vi "Periodic Tasks.vi"(8 "error in":errorcluster) -> ()   [LabVIEW 2016]
doc: "This VI runs in parallel to other tasks. It can contain as many user-defined periodic loops as you need. These can carry out PID or other sorts of timed response."
uses:
  <vilib>/Rock Robotics/WPI/DriverStation/WPI_DriverStationRobotMode2.ctl
  <vilib>/Rock Robotics/WPI/Utilities/WPI_GetSetVariantRefNum.vi
  <vilib>/Rock Robotics/Network Tables/NT Write Number.vi
  <vilib>/Instr/_visa.llb/VISA Configure Serial Port (Instr).vi
  Systems/Global 1.vi
  Global 2.vi
panel:
  out "Waveform Chart":dbl(graph)
  out "PSI":dbl=101.0986199
  out "Shoot 0":dbl format="%#_13g"
  out "Shoot 1":dbl format="%#_13g"
  out "read buffer":string="B:2,X:203.00"
  in  "Search_Params":string[](array[string])=["B", "X", "Y", "W1", "H1", "W2", "H2"]
  out "Last Complete Message":string="B:2,X:203.00,Y:125.00,W1:11,H1:27,W2:8,H2:25"
  out "length":i32=44
  in  "off set":dbl format="%#_13g"
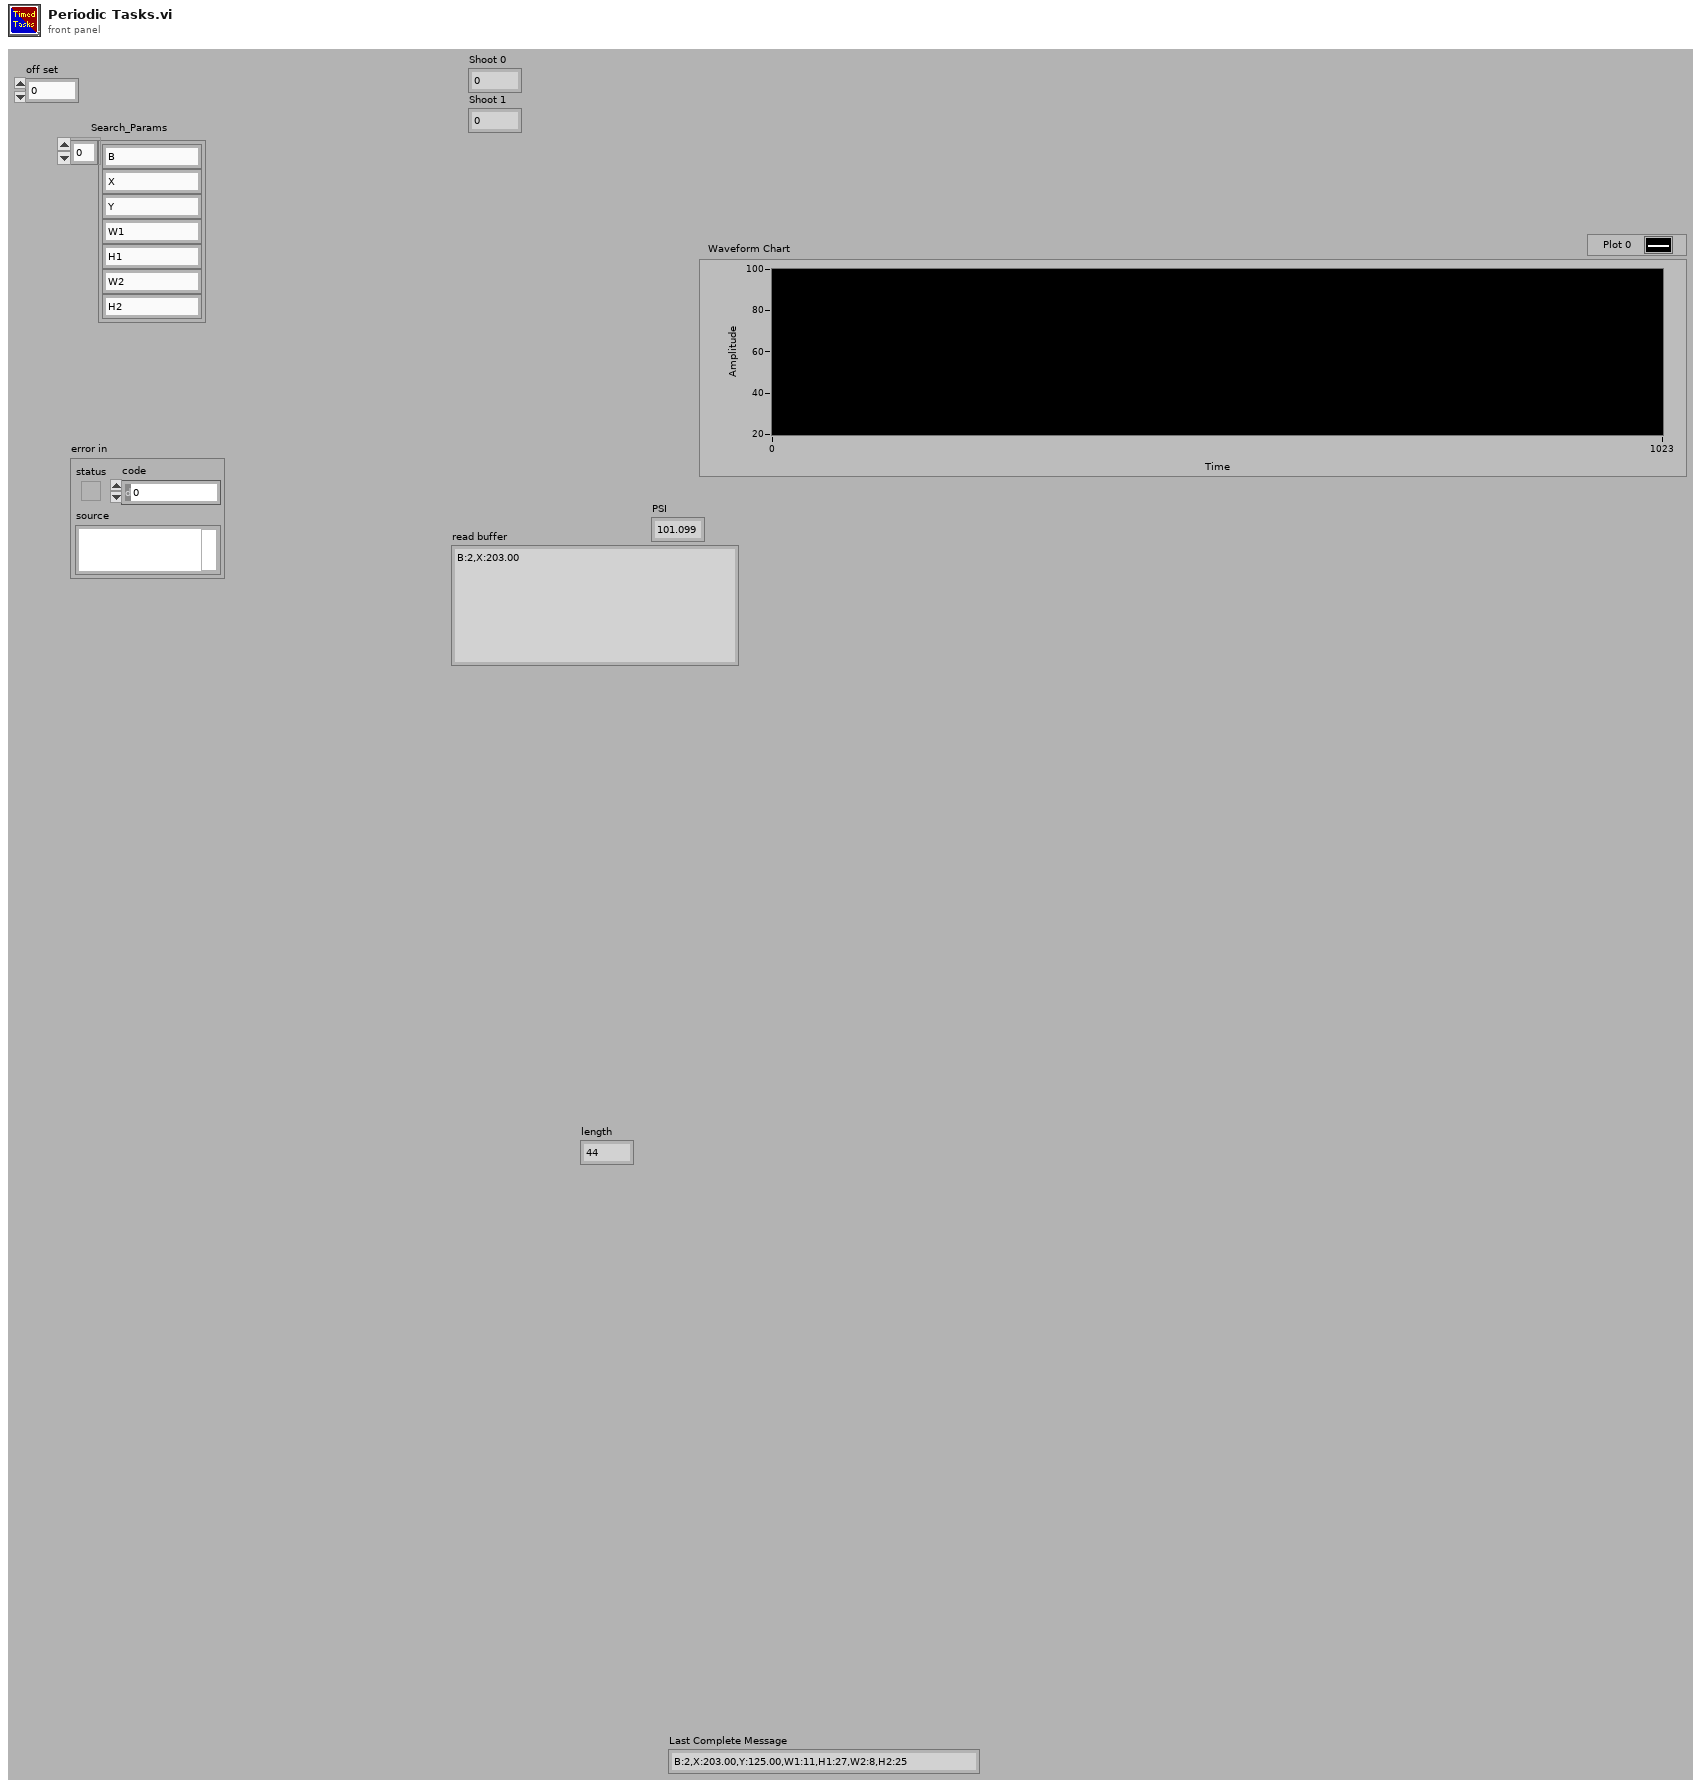
[diagram p1: front panel]
types:
  T1 = typedef "WPI_JoystickDevRef.ctl" = cluster{"Device":T2}
  T2 = typedef "WPI_JoystickDeviceEnum.ctl" = enum16{"USB 0", "USB 1", "USB 2", "USB 3", "USB 4", "USB 5"}
  T3 = typedef "WPI_AnalogChannelDevRef.ctl" = cluster{"DevStatus":errorcluster, "Analog Channel":T4}
  T4 = typedef "FPGA_AIChannel.ctl" = enum8{"AI 0", "AI 1", "AI 2", "AI 3", "AI MXP 0", "AI MXP 1", "AI MXP 2", "AI MXP 3", "Invalid"}
  T5 = typedef "WPI_MotorControlDeviceRef.ctl" = cluster{"DeviceStatus":errorcluster, "Type":T6, "PWM":cluster{"PWM Channel":T7, "DeadBand":T8}, "CAN":cluster{"Device Number":u8, "SetOutput VI Ref":variant, "GetOutput VI Ref":variant, "Enable VI Ref":variant, "Disable VI Ref":variant, "Data":variant}, "Invert":bool}
  T6 = typedef "WPI_MotorControlType.ctl" = enum16{"PWM", "CAN"}
  T7 = typedef "FPGA_DIOPWMChannel.ctl" = enum8{"PWM 0", "PWM 1", "PWM 2", "PWM 3", "PWM 4", "PWM 5", "PWM 6", "PWM 7", "PWM 8", "PWM 9", "PWM MXP 0", "PWM MXP 1", "PWM MXP 2", "PWM MXP 3", "PWM MXP 4", "PWM MXP 5", "PWM MXP 6", "PWM MXP 7", "PWM MXP 8", "PWM MXP 9", "Invalid"}
  T8 = typedef "WPI_PWMDeadband.ctl" = cluster{"Name":string, "maxPositivePwm":i32, "minPositivePwm":i32, "centerPwm":i32, "maxNegativePwm":i32, "minNegativePwm":i32, "angularRange":u16}
  T9 = typedef "WPI_DriverStationRobotMode2.ctl" = enum16{"Autonomous Disabled", "Autonomous Enabled", "Teleop Disabled", "Teleop Enabled", "Disconnected", "Finish", "Test Disabled", "Test Enabled", "Emergency Stopped"}
  T10 = typedef "WPI_CANTalonSRX_GlobalStatus.ctl" = cluster{"Applied Throttle":dbl, "Module Enabled":bool, "CAN Error":errorcluster, "Closed Loop Error":dbl, "Forward Limit Switch Closed":bool, "Reverse Limit Switch Closed":bool, "Sensor Position":dbl, "Sensor Velocity":dbl, "Current":dbl, "Sticky Fault - Over Temp":bool, "Sticky Fault - Under Voltage":bool, "Sticky Fault - Forward Limit":bool, "Sticky Fault - Reverse Limit":bool, "Sticky Fault - Forward Soft Limit":bool, "Sticky Fault - Reverse Soft Limit":bool, "Brake is Enabled":bool, "Encoder Position":dbl, "Encoder Velocity":dbl, "Encoder Index Count":dbl, "Encoder A Pin State":bool, "Encoder B Pin State":bool, "Encoder Index Pin State":bool, "Analog In":dbl, "Analog In Velocity":dbl, "Temperature (C)":dbl, "Battery Voltage":dbl, "Control 5 Is Supported":bool, "Current Profile Slot Select":dbl, "Pos Div 8":bool, "Vel Div 4":bool, "Pulse Width Position":i32, "Pulse Width Velocity":i32, "Pulse Width Rise To Rise (us)":i32, "Pulse Width Rise To Fall (us)":i32, "Mot Prof Active Is Under Run":bool, "Mot Prof Active Has Under Run":bool, "Mot Prof Active Is Last":bool, "Mot Prof Active Velocity Only":bool, "Mot Prof Active Is Valid":bool, "Mot Prof Buffer Is Full":bool, "Mot Prof Active Profile Slot Select":i32, "Mot Prof NextID":i32, "Mot Prof Count":i32, "Mot Prof Active Velocity":dbl, "Mot Prof Active Position":dbl, "Mot Prof Output Enable":i32}
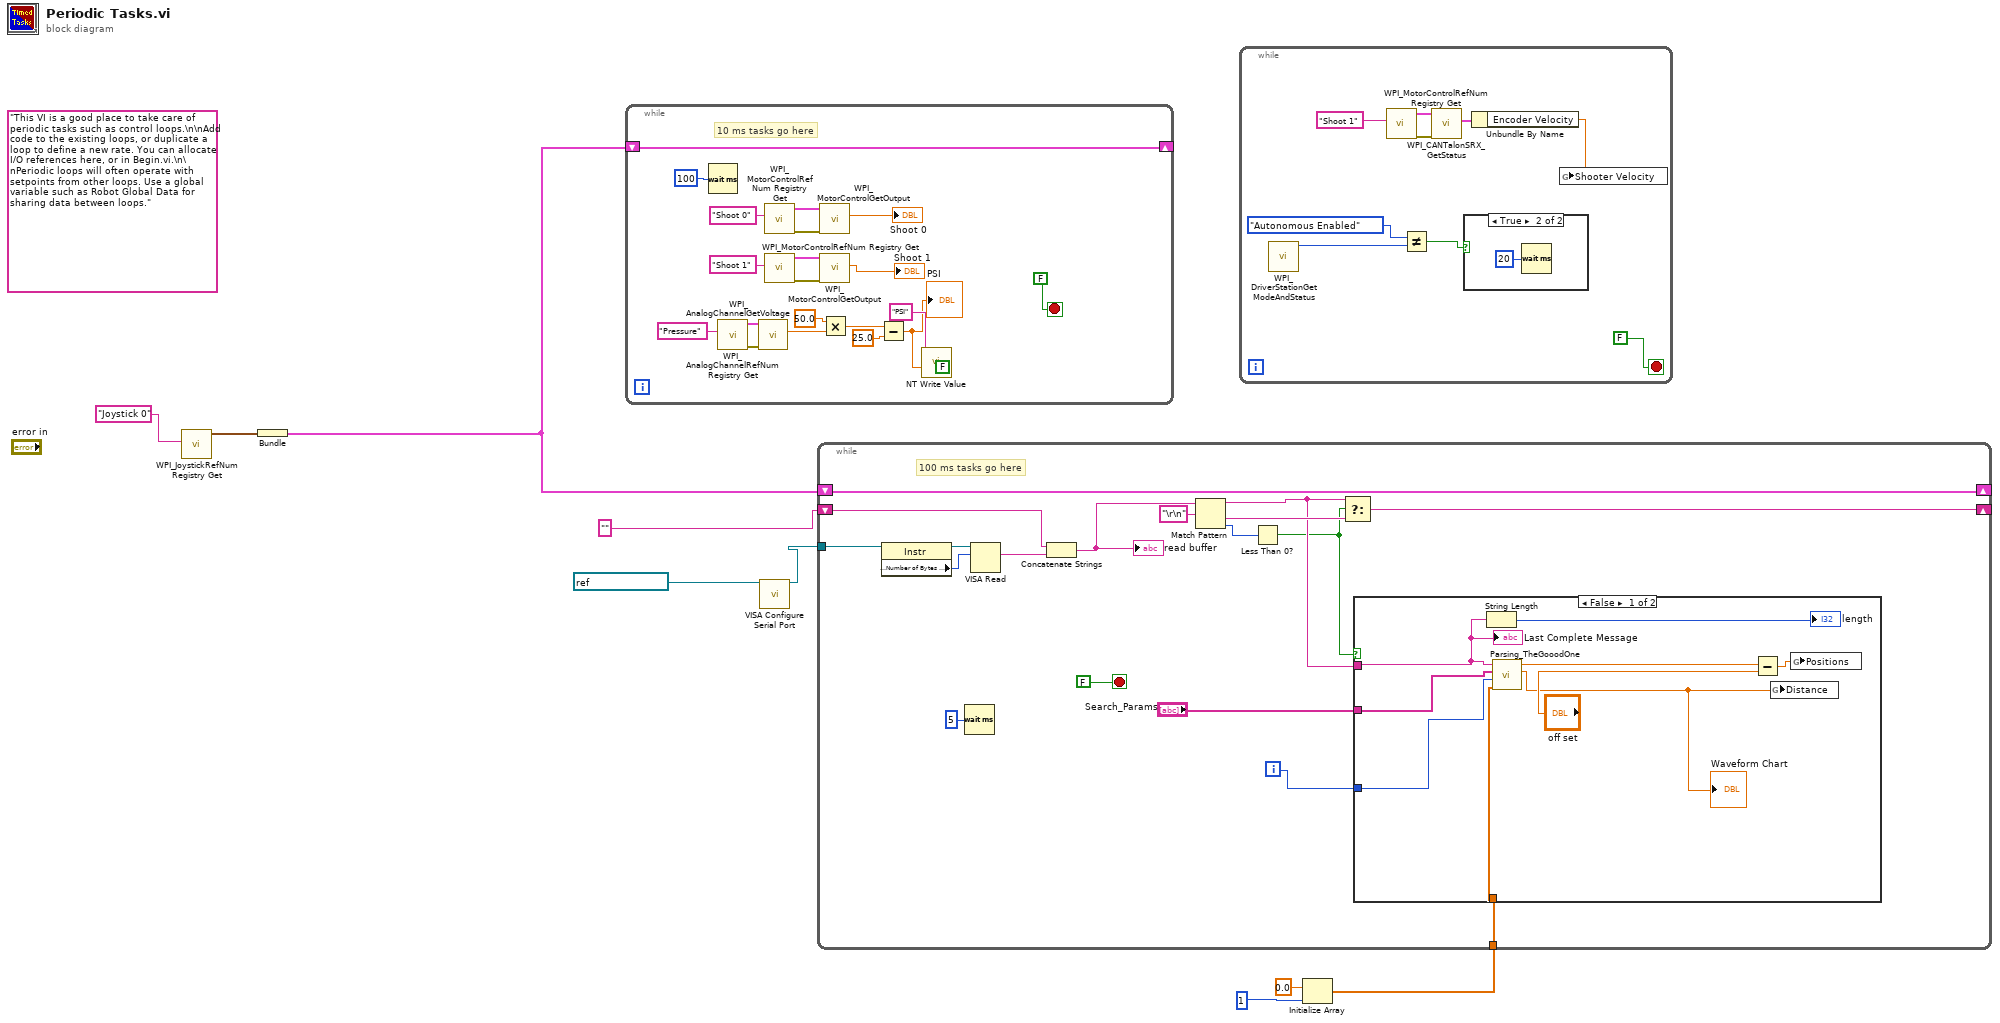
[diagram p0: block diagram]
diagram:
  (unwired) "This VI is a good place to take care of periodic tasks such as control loops.\n\nAdd code to the existing loops, or duplicate a loop to define a new rate. You can allocate I/O references here, or in Begin.vi.\n\nPeriodic loops will often operate with setpoints from other loops. Use a global variable such as Robot Global Data for sharing data between loops."
  n1 = call <vilib>:"WPI_JoystickRefNum Registry Get.vi"("refnum name"="Joystick 0") -> ("JoystickDevRef"=w2:T1)  [unwired: 1 in, 9 out]
  n2 = Bundle("JoystickDevRef"=w2) -> (w3:cluster{"JoystickDevRef":T1})  [unwired: 1 out]
  n3 = while {
    shift-right: [w27] -> _
    shift-left: w3 -> [w27]
    stop <- FALSE stop-if-true
    (unwired) FALSE
    # "10 ms tasks go here"
    n4 = Wait (ms)(milliseconds to wait=u32 100) -> ()  [unwired: 1 out]
    n5 = call <vilib>:"WPI_AnalogChannelRefNum Registry Get.vi"("refnum name"="Pressure") -> ("error out"=w18:errorcluster, "AIDeviceRef"=w17:T3)  [unwired: 9 in]
    n6 = call <vilib>:"WPI_AnalogChannelGetVoltage.vi"("error in (no error)"=w18, "AIDeviceRef"=w17) -> ("Voltage"=w15:dbl)  [unwired: 7 in, 2 out]
    n7 = call <vilib>:"WPI_MotorControlRefNum Registry Get.vi"("refnum name"="Shoot 0") -> ("error out"=w22:errorcluster, "MotorControlDevRef"=w26:T5)  [unwired: 9 in]
    n8 = call <vilib>:"WPI_MotorControlRefNum Registry Get.vi"("refnum name"="Shoot 1") -> ("error out"=w21:errorcluster, "MotorControlDevRef"=w23:T5)  [unwired: 9 in]
    n9 = call <vilib>:"WPI_MotorControlGetOutput.vi"("error in"=w22, "MotorControlDevRef"=w26) -> ("Output"=→"Shoot 0":dbl)  [unwired: 7 in, 2 out]
    n10 = call <vilib>:"WPI_MotorControlGetOutput.vi"("error in"=w21, "MotorControlDevRef"=w23) -> ("Output"=→"Shoot 1":dbl)  [unwired: 7 in, 2 out]
    n11 = Multiply(x=50.0, y=w15) -> (x*y=w13:dbl)
    n12 = Subtract(x=w13, y=25.0) -> (x-y=w10:dbl)
    "PSI" <- w10
    n13 = call-poly <vilib>:"NT Write Value.vi"("Numeric"=w10, "Name"="PSI") -> ()  [unwired: 9 in, 1 out]
  }
  n14 = call-poly "VISA Configure Serial Port"("VISA resource name"=refnum<visa-resource-name> "ASRL2::INSTR") -> ("VISA resource name out"=w5:refnum<visa-resource-name>)  [unwired: 13 in, 1 out]
  n15 = while {
    stop <- FALSE stop-if-true
    n16 = call <vilib>:"WPI_DriverStationGetModeAndStatus.vi"() -> ("Robot Mode"=w32:T9)  [unwired: 10 in, 1 out]
    n17 = call <vilib>:"WPI_MotorControlRefNum Registry Get.vi"("refnum name"="Shoot 1") -> ("error out"=w36:errorcluster, "MotorControlDevRef"=w37:T5)  [unwired: 9 in]
    n18 = Not Equal?(x=WPI_DriverStationRobotMode2."Autonomous Enabled" ("Robot Mode"), y=w32) -> (x != y?=w30:bool)
    n19 = call <vilib>:"WPI_CANTalonSRX_GetStatus.vi"("error in (no error)"=w36, "CAN Talon SRX Ref"=w37) -> ("Talon SRX Status"=w35:T10)  [unwired: 7 in, 2 out]
    n20 = case shown="True" w30 {
      frame False {
      }
      frame True {
        n21 = Wait (ms)(milliseconds to wait=u32 20) -> ()  [unwired: 1 out]
      }
    }
    n22 = Unbundle By Name(w35) -> ("Encoder Velocity"=w34:dbl)
    n23 = global write "Global 2.vi" "Shooter Velocity"(w34) -> ()
  }
  n24 = Initialize Array(0.0 ("element"), 1) -> (w9:dbl[])
  n25 = while {
    shift-right: [w56] -> _
    shift-left: w3 -> [w56]
    tunnel: w5 -> [w51]
    shift-right: [w43] -> _
    shift-left: "" -> [w50]
    tunnel: w9 -> [w40]
    i -> [w41]
    stop <- FALSE stop-if-true
    # "100 ms tasks go here"
    n26 = property class="Instr"(reference=w51) -> (reference out=w55:refnum<visa-resource-name>, "Serial Settings:Number of Bytes at Serial Port"=w54:u32)  [unwired: 1 in, 1 out]
    n27 = Wait (ms)(milliseconds to wait=u32 5) -> ()  [unwired: 1 out]
    n28 = VISA Read(VISA resource name=w55, byte count=w54) -> (read buffer=w49:string)  [unwired: 1 in, 3 out]
    n29 = Concatenate Strings(w50, w49) -> (w48:string)
    "read buffer" <- w48
    n30 = Match Pattern(string=w48, regular expression="\r\n") -> (before substring=w44:string, after substring=w45:string, offset past match=w46:i32)  [unwired: 1 in, 1 out]
    n31 = Less Than 0?(x=w46) -> (x < 0?=w42:bool)
    n32 = Select(t=w44, s=w42, f=w45) -> (s? t:f=w43:string)
    n33 = case shown="False" w42 {
      tunnel: "Search_Params" -> [w65 _]
      tunnel: w44 -> [w64 _]
      tunnel: w41 -> [w60 _]
      tunnel: w40 -> [w59 _]
      frame False {
        n34 = String Length(string=w64) -> (length=→"length":i32)
        n35 = call "Parsing_TheGooodOne.vi"("array"=w59, "Iterations"=w60, "Search_Params"=w65, "Input"=w64) -> ("Corrected distance"=w58:dbl, "Value-Reference"=w63:dbl)  [unwired: 4 in]
        "Waveform Chart" <- w58
        n36 = Subtract(x=w63, y="off set") -> (x-y=w61:dbl)
        n37 = global write "Global 1.vi" "Distance"(w58) -> ()
        n38 = global write "Global 1.vi" "Positions"(w61) -> ()
        "Last Complete Message" <- w64
      }
      frame True {
      }
    }
  }
